vi "ziModExecuteTimeout.vi"(7 "Error In":errorcluster, 8 "Timeout 5000ms":u32=5000, 9 "Modal (F)":bool, 10 "ziModHandle In":T1 {"ModHandle" format="0x%08x"; "Conn" format="0x%08x"}) -> (0 "Error Out":errorcluster, 2 "Finished?":bool, 3 "ziModHandle Out":T1 {"ModHandle" format="0x%08x"; "Conn" format="0x%08x"})   [LabVIEW 2009, in "Zurich Instruments LabOne.lvlib"]
doc: "Start the module. If the <b>Modal</b> is set to false, the vi waits for the module to finish and polls the data from the device. Use ziModGetNextNode.vi in order to access the availible data. If the <b>Modal</b> is set to true, the module is started. In order to poll the data from the device use ziModRead.vi."
uses:
  <instrlib>/Zurich Instruments LabOne/Zurich Instruments LabOne.lvlib
  <instrlib>/Zurich Instruments LabOne/Public/Modules/ziTypeModHandle.ctl
  <instrlib>/Zurich Instruments LabOne/Private/ziLV64.dll
panel:
  out "Timeout?":bool
  in  "stop":bool
  out "Progress (unity)":dbl
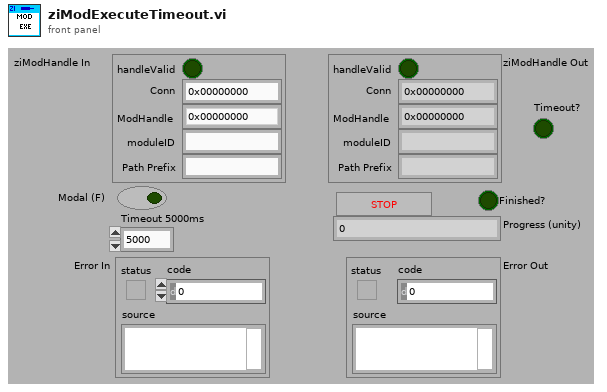
[diagram p1: front panel]
types:
  T1 = typedef "Zurich Instruments LabOne.lvlib/ziTypeModHandle.ctl" = cluster{"handleValid":bool, "Conn":u64, "ModHandle":u64, "moduleID":string, "Path Prefix":string}
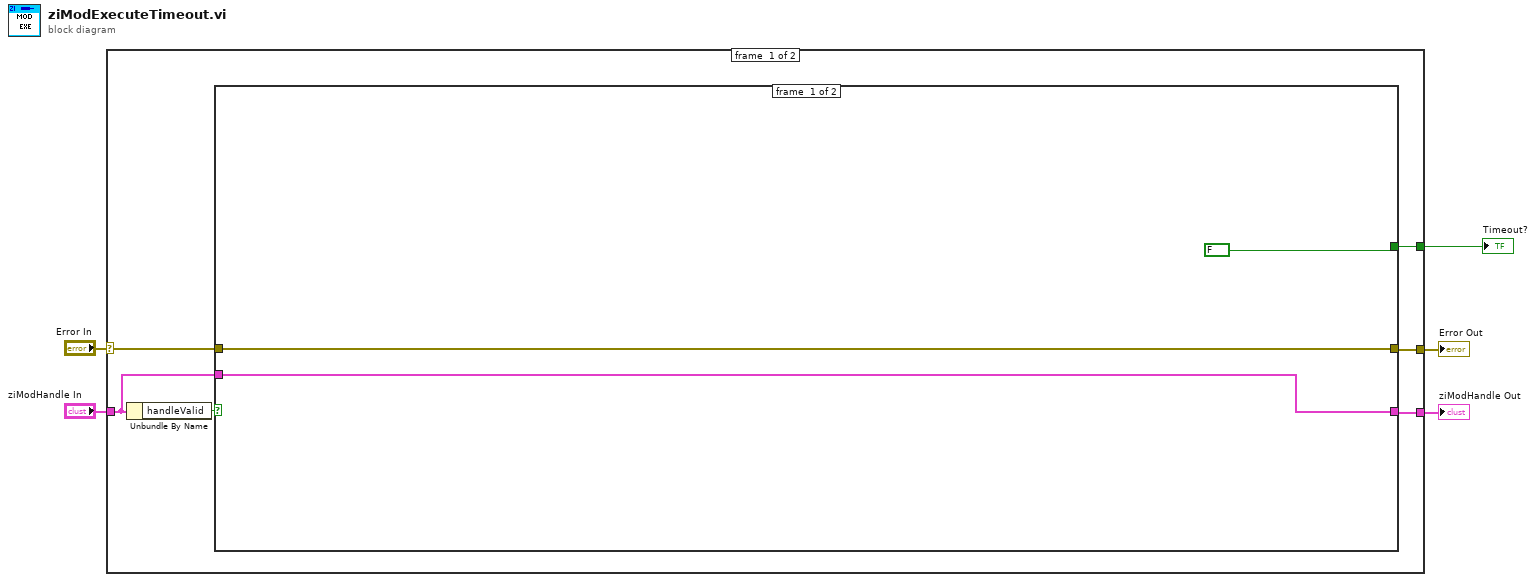
[diagram p0: block diagram]
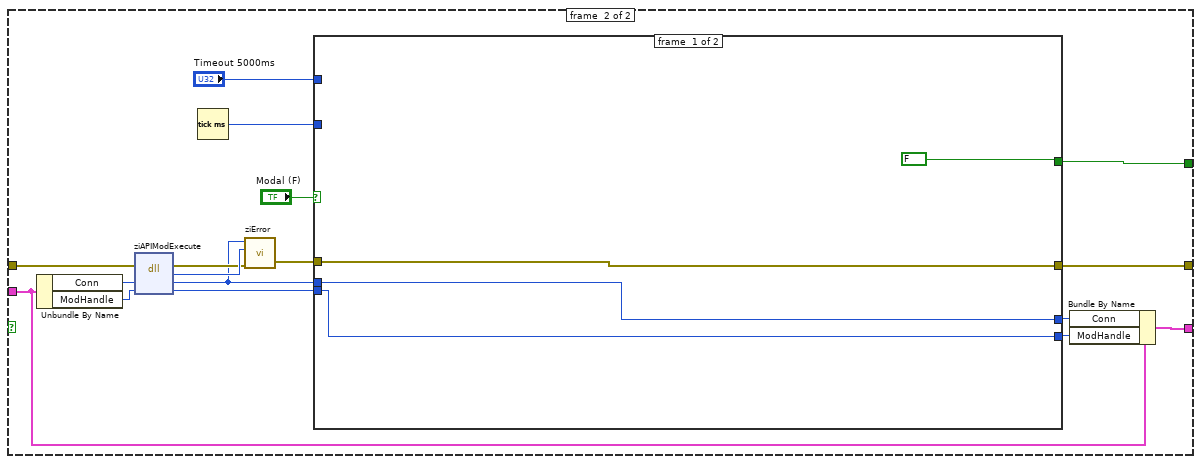
[diagram p2: hidden frame]
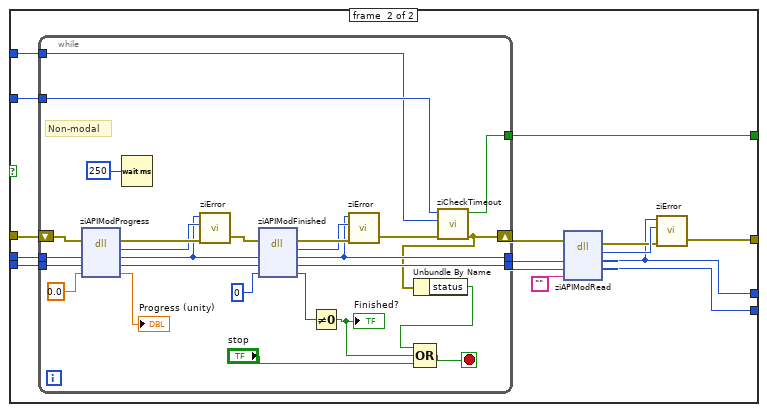
[diagram p3: hidden frame]
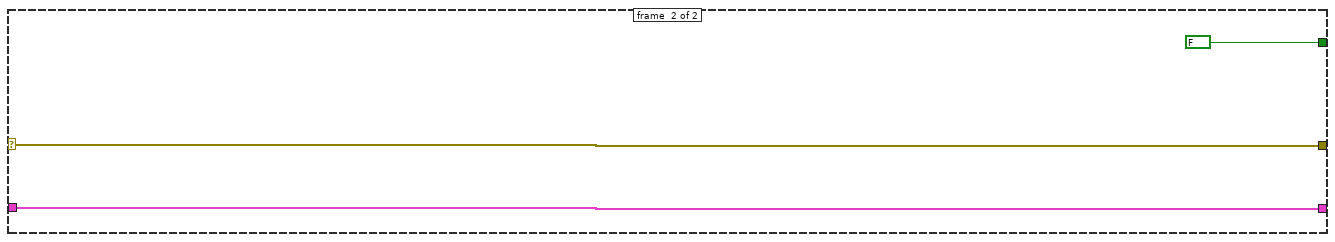
[diagram p4: hidden frame]
diagram:
  n1 = case shown="No Error" "Error In" {
    selector: "Error In" -> [w9 w79]
    tunnel: "ziModHandle In" -> [w8 w78]
    tunnel: [w11 w78] -> w2
    tunnel: [w10 w79] -> w5
    tunnel: [w6 FALSE] -> w1
    frame #0 {
      n2 = Unbundle By Name(w8) -> ("handleValid"=w7:bool)
      n3 = case shown="True" w7 {
        tunnel: w8 -> [w14 w28]
        tunnel: [w14 w27] -> w11
        tunnel: w9 -> [w13 w31]
        tunnel: [w13 w19] -> w10
        tunnel: [FALSE w15] -> w6
        frame #0 {
        }
        frame #1 {
          n4 = Unbundle By Name(w28) -> ("Conn"=w30:u64, "ModHandle"=w29:u64)
          n5 = dll-call lib="C:/Program Files/National Instruments/LabVIEW 2009/instr.lib/Zurich Instruments LabOne/Private/ziLV*.*" fn="ziAPIModExecute"(error in=w31, "conn"=w30, "ModHandle"=w29) -> (error out=w21:errorcluster, "return type"=w22:u32, "conn"=w18:u64, "ModHandle"=w26:u64)  [unwired: 2 in, 1 out]
          n6 = Tick Count (ms)() -> (millisecond timer value=w17:u32)
          n7 = call <instrlib>:"ziError.vi"("Conn"=w18, "ziErrorCode"=w22, "Error In"=w21) -> ("Error Out"=w20:errorcluster)  [unwired: 2 in, 1 out]
          n8 = case shown="False" "Modal (F)" {
            tunnel: w18 -> [w34 w50]
            tunnel: w26 -> [w33 w49]
            tunnel: [w35 w40] -> w19
            tunnel: [w33 w44] -> w25
            tunnel: [w34 w39] -> w24
            tunnel: w20 -> [w35 w43]
            tunnel: w17 -> [_ w38]
            tunnel: "Timeout 5000ms" -> [_ w37]
            tunnel: [FALSE w36] -> w15
            frame #0 {
            }
            frame #1 {
              # "Non-modal"
              n9 = while {
                tunnel: w50 -> [w75]
                tunnel: w49 -> [w74]
                tunnel: [w76] -> w45
                tunnel: [w60] -> w46
                shift-right: [w55] -> w47
                shift-left: w43 -> [w64]
                tunnel: w38 -> [w59]
                tunnel: w37 -> [w58]
                tunnel: [w51] -> w36
                stop <- w56 stop-if-true
                n10 = dll-call lib="C:/Program Files/National Instruments/LabVIEW 2009/instr.lib/Zurich Instruments LabOne/Private/ziLV*.*" fn="ziAPIModProgress"(error in=w64, "conn"=w75, "ModHandle"=w74, "Finished"=0.0) -> (error out=w70:errorcluster, "return type"=w68:u32, "conn"=w61:u64, "ModHandle"=w73:u64, "Finished"=→"Progress (unity)":dbl)  [unwired: 2 in, 1 out]
                n11 = Wait (ms)(milliseconds to wait=u32 250) -> ()  [unwired: 1 out]
                n12 = call <instrlib>:"ziError.vi"("Conn"=w61, "ziErrorCode"=w68, "Error In"=w70) -> ("Error Out"=w69:errorcluster)  [unwired: 2 in, 1 out]
                n13 = dll-call lib="C:/Program Files/National Instruments/LabVIEW 2009/instr.lib/Zurich Instruments LabOne/Private/ziLV*.*" fn="ziAPIModFinished"(error in=w69, "conn"=w61, "ModHandle"=w73, "Finished"=i64 0) -> (error out=w67:errorcluster, "return type"=w66:u32, "conn"=w60:u64, "ModHandle"=w76:u64, "Finished"=w71:i64)  [unwired: 2 in, 1 out]
                n14 = Not Equal To 0?(x=w71) -> (x != 0?=w53:bool)
                "Finished?" <- w53
                n15 = call <instrlib>:"ziError.vi"("Conn"=w60, "ziErrorCode"=w66, "Error In"=w67) -> ("Error Out"=w57:errorcluster)  [unwired: 2 in, 1 out]
                n16 = call <instrlib>:"ziCheckTimeout.vi"("Error In"=w57, "Timeout Value (5000ms)"=w58, "current tick count (ms)"=w59) -> ("Error Out"=w55:errorcluster, "Timeout?"=w51:bool)  [unwired: 7 in]
                n17 = Unbundle By Name(w55) -> ("status"=w52:bool)
                n18 = Compound Arithmetic op=OR(w52, w53, "stop") -> (w56:bool)
              }
              n19 = dll-call lib="C:/Program Files/National Instruments/LabVIEW 2009/instr.lib/Zurich Instruments LabOne/Private/ziLV*.*" fn="ziAPIModRead"(error in=w47, "Conn"=w46, "ModHandle"=w45, "Path"="") -> (error out=w41:errorcluster, "return type"=w42:u32, "Conn"=w39:u64, "ModHandle"=w44:u64)  [unwired: 3 in, 1 out]
              n20 = call <instrlib>:"ziError.vi"("Conn"=w39, "ziErrorCode"=w42, "Error In"=w41) -> ("Error Out"=w40:errorcluster)  [unwired: 2 in, 1 out]
            }
          }
          n21 = Bundle By Name(cluster=w28, "Conn"=w24, "ModHandle"=w25) -> (w27:T1)
        }
      }
    }
    frame #1 {
    }
  }
  "Error Out" <- w5
  "ziModHandle Out" <- w2
  "Timeout?" <- w1
